vi "Method.vi"(4 "Input B":refnum<class "Abs_Numeric.lvclass">, 5 "Input A":T1) -> (1 "Result":T1)   [LabVIEW 2021, in "Multiply_U64.lvclass"]
uses:
  Multiply_U64.lvclass
  Abs_Type.ctl
  Abs_Types/U64 Integer/Abs_U64 Integer.lvclass
  Abs_Types/Numeric/Abs_Numeric.lvclass
  C:/Users/Tim/Documents/LabVIEW/2021/Data Classes/Source/Functions/Support/Two Terminal/U64/AbsFunc_Two Term_U64.lvclass
  C:/Users/Tim/Documents/LabVIEW/2021/Data Classes/Source/Abs_Types/U64 Integer/Abs_U64 Integer.lvclass
  Support/Two Terminal/U64/AbsFunc_Two Term_U64.lvclass/AbsFunc_Two Term_U64.ctl
  Support/Two Terminal/U64/Properties/Write Numeric A.vi
  Support/Two Terminal/U64/Properties/Write Numeric B.vi
  Multiply_U64.lvclass/Multiply_U64.ctl
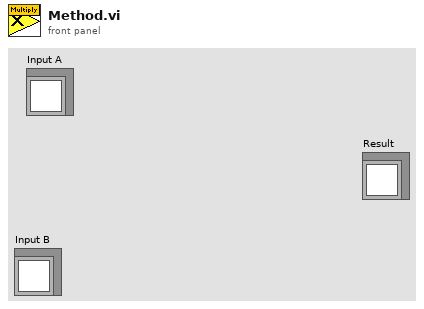
[diagram p1: front panel]
types:
  T1 = typedef "Multiply_U64.lvclass/Abs_Type.ctl" = refnum<class "Abs_U64 Integer.lvclass">
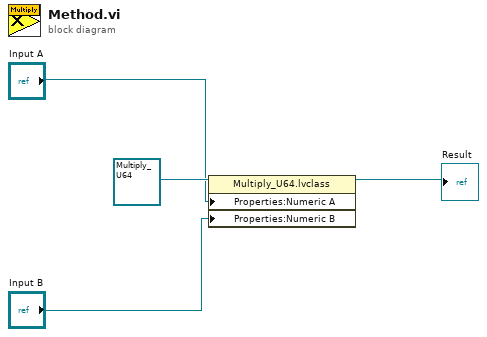
[diagram p0: block diagram]
diagram:
  n1 = property class="Multiply_U64.lvclass"(reference=refnum<class "Multiply_U64.lvclass"> refnum ("Functions.lvlib:Numeric.lvlib:Multiply.lvclass"), "Properties:Numeric A"="Input A", "Properties:Numeric B"="Input B") -> (reference out=→"Result":refnum<class "Multiply_U64.lvclass">)  [unwired: 1 in, 1 out]
